vi "Save Subsystem Configuration.vi"(8 "error in (no error)":errorcluster, 10 "Subsystems":T1[](array[typedef]), 11 "Configuration Refnum In":T2) -> (0 "error out":errorcluster, 3 "Configuration Refnum Out":T2)   [LabVIEW 2024]
doc: "Saves subsystem configurations."
uses:
  <vilib>/Utility/config.llb/Config Data RefNum.ctl
  Controls/Server/Subsystem Configuration.ctl
  <vilib>/Utility/config.llb/Write Key (String).vi
  <vilib>/Utility/config.llb/NI_LVConfig.lvlib
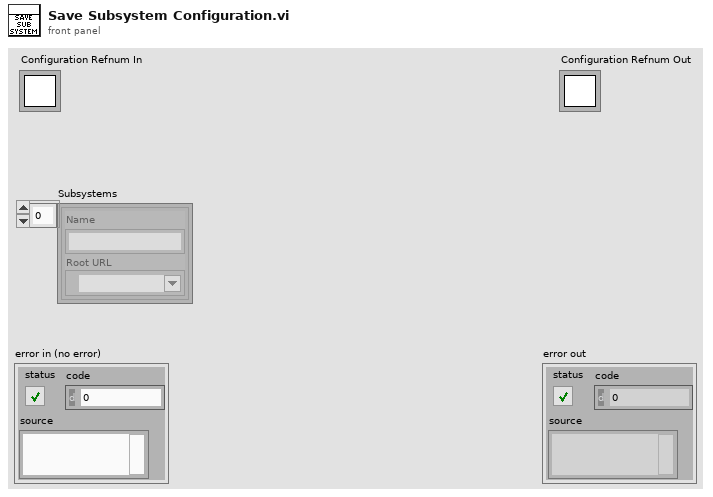
[diagram p1: front panel]
types:
  T1 = typedef "Subsystem Configuration.ctl" = cluster{"Name":string, "Root URL":refnum<k21>}
  T2 = typedef "NI_LVConfig.lvlib/Config Data RefNum.ctl" = refnum<k1>
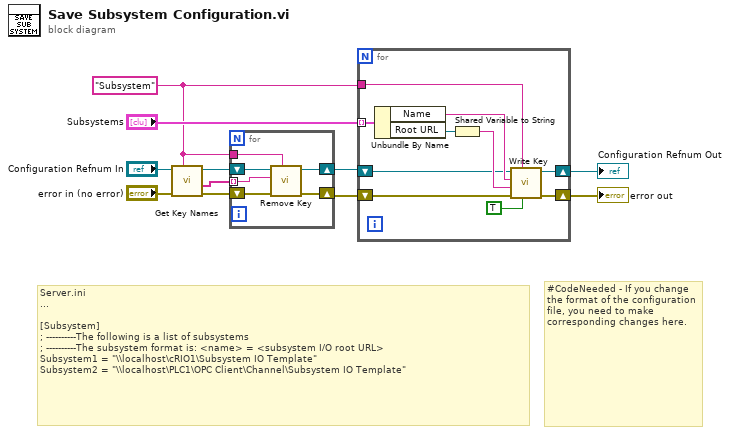
[diagram p0: block diagram]
diagram:
  w3 = "Subsystem" ("section")
  # "#CodeNeeded - If you change the format of the configuration file, you need to make corresponding changes here."
  # "Server.ini\n...\n\n[Subsystem]\n; ----------The following is a list of subsystems\n; ----------The subsystem format is: <name> = <subsystem I/O root URL>\nSubsystem1 = \"\\\\localhost\\cRIO1\\Subsystem IO Template\"\nSubsystem2 = \"\\\\localhost\\PLC1\\OPC Client\\Channel\\Subsystem IO Template\""
  n1 = call <vilib>:"Get Key Names.vi"("section"=w3, "error in (no error)"="error in (no error)", "refnum"="Configuration Refnum In") -> ("error out"=w6:errorcluster, "key names"=w7:string[], "refnum out"=w8:T2)  [unwired: 5 in, 1 out]
  n2 = for {
    shift-right: [w17] -> w4
    shift-left: w6 -> [w14]
    shift-right: [w16] -> w5
    shift-left: w8 -> [w15]
    tunnel: w7 -> [w13] mode=indexing
    tunnel: w3 -> [w12]
    n3 = call <vilib>:"Remove Key.vi"("section"=w12, "error in (no error)"=w14, "key"=w13, "refnum"=w15) -> ("error out"=w17:errorcluster, "refnum out"=w16:T2)  [unwired: 5 in, 1 out]
  }
  n4 = for {
    shift-right: [w27] -> w11
    shift-left: w5 -> [w20]
    shift-right: [w26] -> w10
    shift-left: w4 -> [w19]
    tunnel: "Subsystems" -> [w22] mode=indexing
    tunnel: w3 -> [w21]
    n5 = Unbundle By Name(w22) -> ("Name"=w25:string, "Root URL"=w24:refnum<k21>)
    n6 = Shared Variable to String(1:w24) -> (0:w23:string)
    n7 = call-poly <vilib>:"Write Key.vi"("write raw string? (F)"=TRUE, "section"=w21, "error in (no error)"=w19, "value"=w23, "key"=w25, "refnum"=w20) -> ("error out"=w26:errorcluster, "refnum out"=w27:T2)  [unwired: 3 in, 1 out]
  }
  "error out" <- w10
  "Configuration Refnum Out" <- w11
